vi "Opis predmeta.vi"(2 "Enum":T1(ring)=enum."CEKAJ", 3 "PREDMET":enum16{"A", "B", "C"}(ring)) -> (0 "Enum 2":T1(ring), 1 "Opis predmeta":T2)   [LabVIEW 2017]
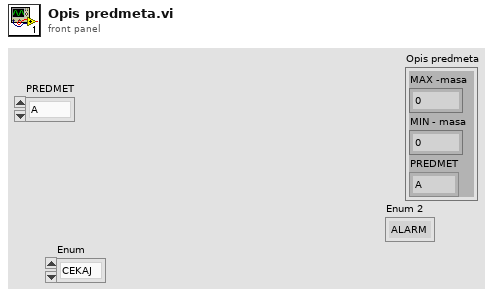
[diagram p1: front panel]
types:
  T1 = enum16{"ALARM", "IZABERI", "CEKAJ", "MERENJE", "POKRENI", "SLIKANJE"}
  T2 = cluster{"MAX -masa":dbl, "MIN - masa":dbl, "PREDMET":enum16{"A", "B", "C"}}
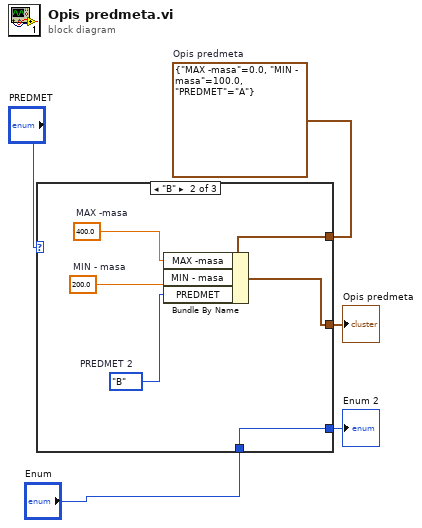
[diagram p0: block diagram]
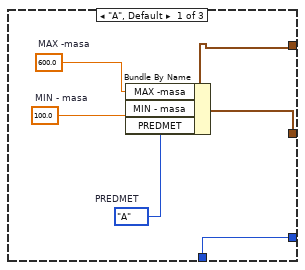
[diagram p2: hidden frame]
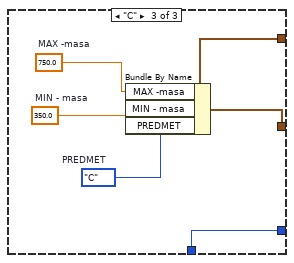
[diagram p3: hidden frame]
diagram:
  w4 = T2 {"MAX -masa"=0.0, "MIN - masa"=100.0, "PREDMET"=enum."A"}  # Opis predmeta
  n1 = case shown="\"B\"" "PREDMET" {
    tunnel: w4 -> [w8 w14 w20]
    tunnel: [w11 w15 w21] -> w3
    tunnel: "Enum" -> [w6 w12 w18]
    tunnel: [w6 w12 w18] -> w1
    frame "A", Default {
      w7 = enum16{"A", "B", "C"}."A"  # PREDMET
      w10 = 600.0  # MAX -masa
      w9 = 100.0  # MIN - masa
      n2 = Bundle By Name(cluster=w8, "MAX -masa"=w10, "MIN - masa"=w9, "PREDMET"=w7) -> (w11:T2)
    }
    frame "B" {
      w13 = enum16{"A", "B", "C"}."B"  # PREDMET 2
      w17 = 400.0  # MAX -masa
      w16 = 200.0  # MIN - masa
      n3 = Bundle By Name(cluster=w14, "MAX -masa"=w17, "MIN - masa"=w16, "PREDMET"=w13) -> (w15:T2)
    }
    frame "C" {
      w19 = enum16{"A", "B", "C"}."C"  # PREDMET
      w23 = 750.0  # MAX -masa
      w22 = 350.0  # MIN - masa
      n4 = Bundle By Name(cluster=w20, "MAX -masa"=w23, "MIN - masa"=w22, "PREDMET"=w19) -> (w21:T2)
    }
  }
  "Opis predmeta" <- w3
  "Enum 2" <- w1
